vi "StopSerial.vi"(8 "error in (no error)":errorcluster, 11 "VISA Refnum in":refnum<visa-resource-name>) -> ()   [LabVIEW 2014, in "Manipulator.lvclass"]
uses:
  Manipulator.lvclass
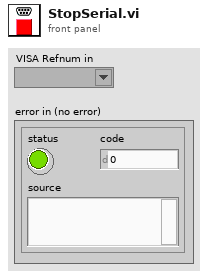
[diagram p1: front panel]
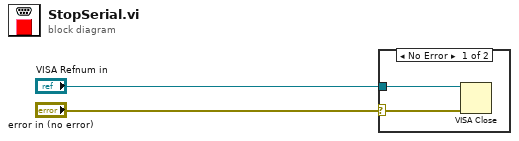
[diagram p0: block diagram]
diagram:
  n1 = case shown="No Error" "error in (no error)" {
    selector: "error in (no error)" -> [w3 _]
    tunnel: "VISA Refnum in" -> [w4 _]
    frame No Error {
      n2 = VISA Close(VISA resource name=w4, error in (no error)=w3) -> ()  [unwired: 1 out]
    }
    frame Error {
    }
  }
